vi "Security.DLL.vi"(8 "error in (no error)":errorcluster, 9 "Option":u8=1, 10 "Seed":u8[](array[numeric])=[254, 233, 229] format="%.0x", 11 "path in":path) -> (0 "error out":errorcluster, 2 "lockstatus":u8, 3 "unsigned byte array":u8[](array[numeric]) format="%.0x")   [LabVIEW 2024, in "Diagnostics Addon Engine.lvlib"]
doc: "extern void __stdcall SecCalcKey(unsigned char *,\n unsigned char, unsigned char,\n unsigned char, unsigned char,\n unsigned char *);"
uses:
  Diagnostics Addon Engine.lvlib
panel:
  out "ucKeyLen":u8[](array[numeric])
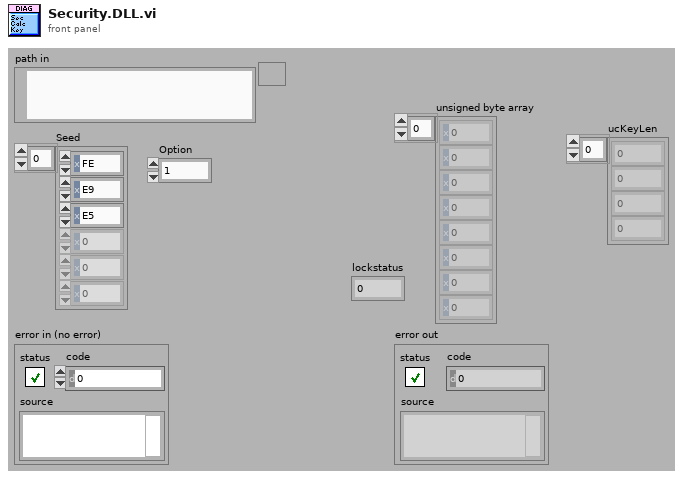
[diagram p1: front panel]
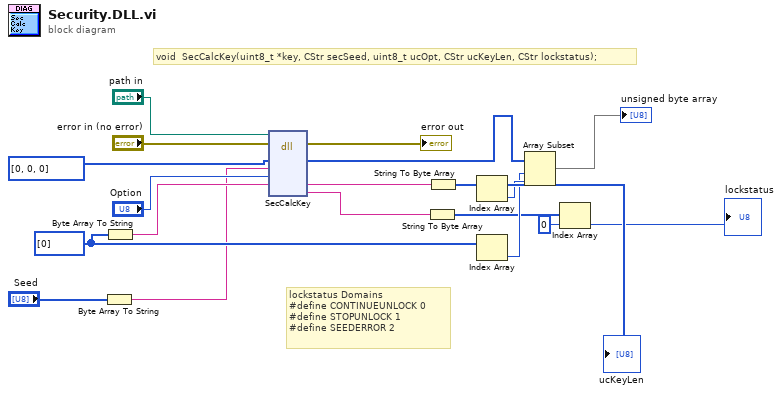
[diagram p0: block diagram]
diagram:
  w17 = u8[] [0] ("unsigned byte array")
  # "lockstatus Domains\n#define CONTINUEUNLOCK 0\n#define STOPUNLOCK 1\n#define SEEDERROR 2"
  # "void  SecCalcKey(uint8_t *key, CStr secSeed, uint8_t ucOpt, CStr ucKeyLen, CStr lockstatus);"
  n1 = Byte Array To String(unsigned byte array="Seed") -> (string=w8:string)
  n2 = Byte Array To String(unsigned byte array=w17) -> (string=w15:string)
  n3 = dll-call lib="C:/_SPDJB/SecKeySPDJB/SecCalcKey.dll" fn="SecCalcKey"(path in="path in", error in="error in (no error)", "key"=u8[] [0, 0, 0] ("unsigned byte array"), "secSeed"=w8, "ucOpt"="Option", "ucKeyLen"=w15) -> (error out=→"error out":errorcluster, "key"=w2:u8[], "ucKeyLen"=w10:string, "lockstatus"=w6:string)  [unwired: 5 in, 1 out]
  n4 = String To Byte Array(string=w6) -> (unsigned byte array=w5:u8[])
  n5 = String To Byte Array(string=w10) -> (unsigned byte array=w19:u8[])
  "ucKeyLen" <- w19
  n6 = Index Array(array=w19) -> (element=w18:u8)  [unwired: 1 in]
  n7 = Index Array(array=w17) -> (element=w16:u8)  [unwired: 1 in]
  n8 = Array Subset(array=w2, index=w16, length=w18) -> (→"unsigned byte array":u8[])
  n9 = Index Array(array=w5, index=0) -> (element=→"lockstatus":u8)
